vi "Test Matrix Copy.vi"() -> ()   [LabVIEW 2014, in "Arduino MatrixMath.lvlib"]
uses:
  Arduino MatrixMath.lvlib
panel:
  out "A copy":sgl[](array[numeric])
  in  "A":sgl[](array[numeric])
  out "Error Out":errorcluster
  in  "Error In":errorcluster
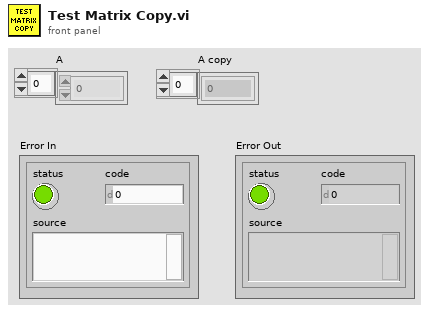
[diagram p1: front panel]
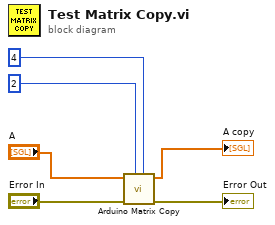
[diagram p0: block diagram]
diagram:
  n1 = call "Arduino Matrix Copy.vi"("cols num."=u8 4, "rows num."=u8 2, "Error In"="Error In", "A"="A") -> ("Error Out"=→"Error Out":errorcluster, "A copy"=→"A copy":sgl[])  [unwired: 6 in]
